vi "Calculate Forward Movement.vi"(8 "Camera Speed":sgl, 9 "Rotation":sgl, 10 "Previous Left":sgl, 11 "Previous Forward":sgl) -> (2 "Next Left":sgl, 3 "Next Forward":sgl)   [LabVIEW 2020, in "Scene.lvclass"]
uses:
  Scene.lvclass
  Scene.lvclass/Scene.ctl
  Graphics/Libraries/3D/3D.lvlib
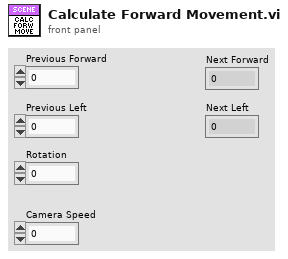
[diagram p1: front panel]
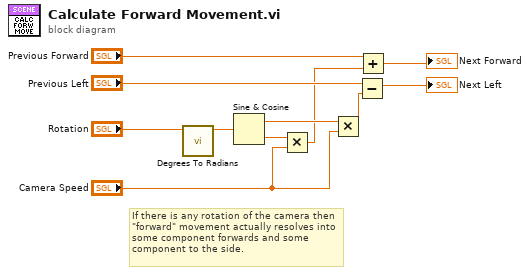
[diagram p0: block diagram]
diagram:
  # "If there is any rotation of the camera then \"forward\" movement actually resolves into some component forwards and some component to the side."
  n1 = call "Degrees To Radians.vi"("Angle (°)"="Rotation") -> ("Angle (rad)"=w7:sgl)  [unwired: 10 in]
  n2 = Sine & Cosine(0:w7) -> (1:w6:sgl, 2:w3:sgl)
  n3 = Multiply(x=w3, y="Camera Speed") -> (x*y=w1:sgl)
  n4 = Multiply(x=w6, y="Camera Speed") -> (x*y=w5:sgl)
  n5 = Subtract(x="Previous Left", y=w5) -> (x-y=→"Next Left":sgl)
  n6 = Add(x="Previous Forward", y=w1) -> (x+y=→"Next Forward":sgl)
